vi "Example Cluster 4.vi"() -> ()   [LabVIEW 2014]
uses:
  ClusterTypedef1.ctl
panel:
  out "Error Out":errorcluster
  in  "Error In":errorcluster
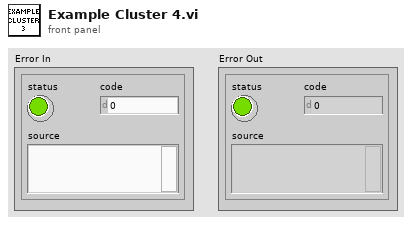
[diagram p1: front panel]
types:
  T1 = typedef "ClusterTypedef1.ctl" = cluster{"some double":dbl}
  T2 = cluster{"numeric_2":i32, "double_2":dbl, "superNestedCluster":T1}
  T3 = cluster{"numeric_1":i32, "double_1":dbl, "superNestedCluster":T1}
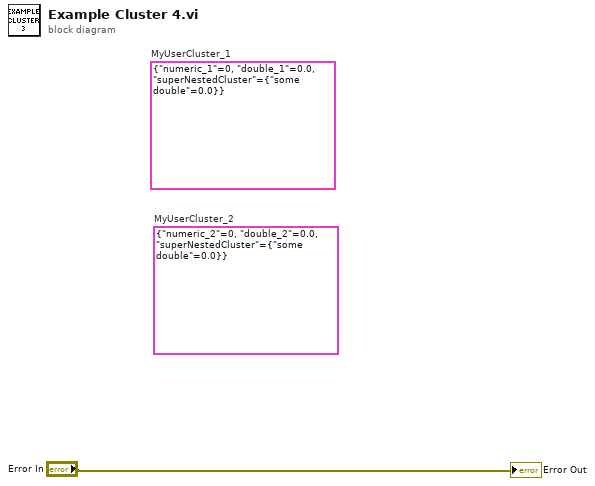
[diagram p0: block diagram]
diagram:
  (unwired) T2 {"numeric_2"=0, "double_2"=0.0, "superNestedCluster"={"some double"=0.0}}  # MyUserCluster_2
  (unwired) T3 {"numeric_1"=0, "double_1"=0.0, "superNestedCluster"={"some double"=0.0}}  # MyUserCluster_1
  "Error Out" <- "Error In"
